vi "Renishaw-XL80_SetExpansionCoefficient.vi"(8 "error in (no error)":errorcluster, 10 "ExpansionCoefficient":dbl, 11 "Renishaw-XL80_EMU in":refnum<class "Renishaw-XL80_EMU.lvclass">) -> (0 "error out":errorcluster, 3 "Renishaw-XL80_EMU out":refnum<class "Renishaw-XL80_EMU.lvclass">)   [LabVIEW 2024, in "Renishaw-XL80_EMU.lvclass"]
doc: "Writing this property will set the material expansion coefficient in ppm/°C.\n\nDefinition\nHRESULTput_ExpansionCoefficient( [in] double newVal);\nParameters\nnewVal\nSpecifies the material expansion coefficient to use in ppm/°C.\n\nComments\nWriting this property always succeeds. It will return an HRESULT of S_OK.\n\nIf the client has set AutoCompensationMode to AUTO_COMPENSATION_FULL then setting this property will also update the material compensation factor."
uses:
  Renishaw-XL80_EMU.lvclass
  Renishaw-XL80_EMU.lvclass/Renishaw-XL80_EMU.ctl
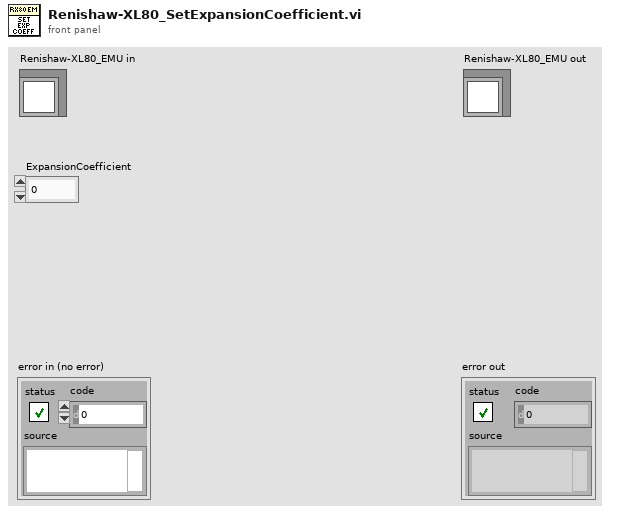
[diagram p1: front panel]
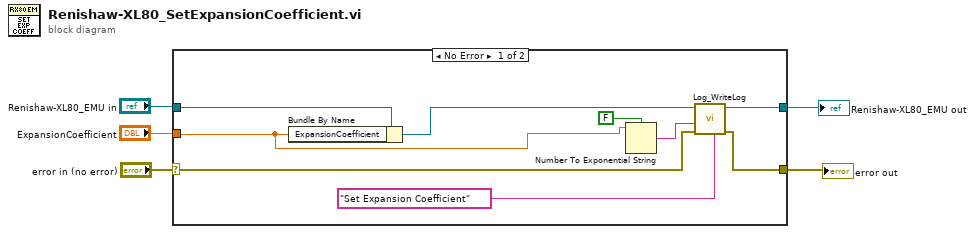
[diagram p0: block diagram]
diagram:
  n1 = case shown="No Error" "error in (no error)" {
    selector: "error in (no error)" -> [w11 w15]
    tunnel: [w12 w16] -> w4
    tunnel: "Renishaw-XL80_EMU in" -> [w14 w16]
    tunnel: [w10 w15] -> w3
    tunnel: "ExpansionCoefficient" -> [w6 _]
    frame No Error {
      n2 = Bundle By Name(cluster=w14, "ExpansionCoefficient"=w6) -> (w13:refnum<class "Renishaw-XL80_EMU.lvclass">)
      n3 = Number To Exponential String(number=w6, 1:FALSE ("use system decimal point (T)")) -> (E-format string=w7:string)  [unwired: 2 in]
      n4 = call-dynamic "Log_WriteLog.vi"("Additional text"="Set Expansion Coefficient", "error in (no error)"=w11, "Response"=w7, "Log in"=w13) -> ("error out"=w10:errorcluster, "Log out"=w12:refnum<class "Renishaw-XL80_EMU.lvclass">)  [unwired: 6 in]
    }
    frame Error {
    }
  }
  "error out" <- w3
  "Renishaw-XL80_EMU out" <- w4
